vi "Sample_process.vi"(8 "Start":i32=20, 9 "Frame number":i32, 11 "Sample data":dbl[](array[numeric])) -> (3 "Image date":dbl[](array[numeric]))   [LabVIEW 2016]
uses:
  <vilib>/Analysis/baseanly.llb/Mean (DBL).vi
  <vilib>/Analysis/NI_AALBase.lvlib
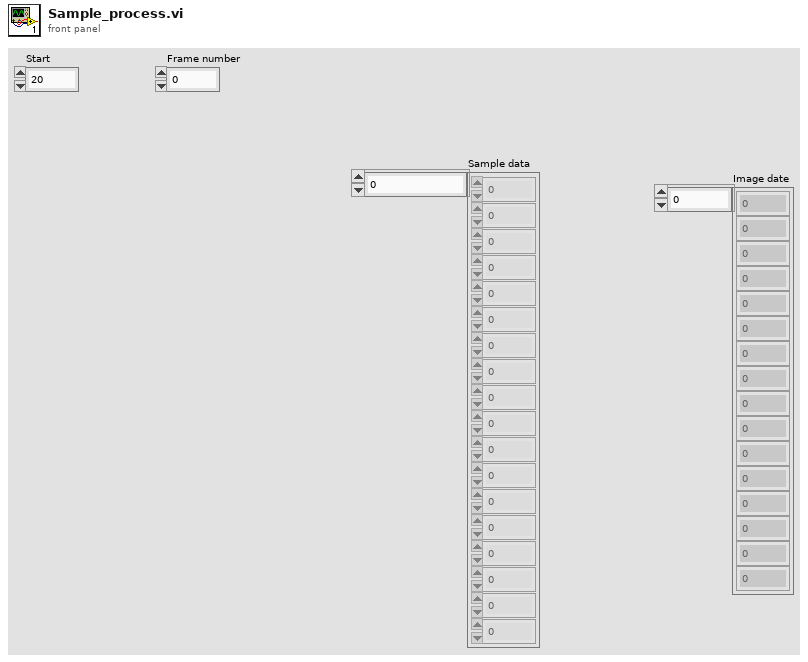
[diagram p1: front panel]
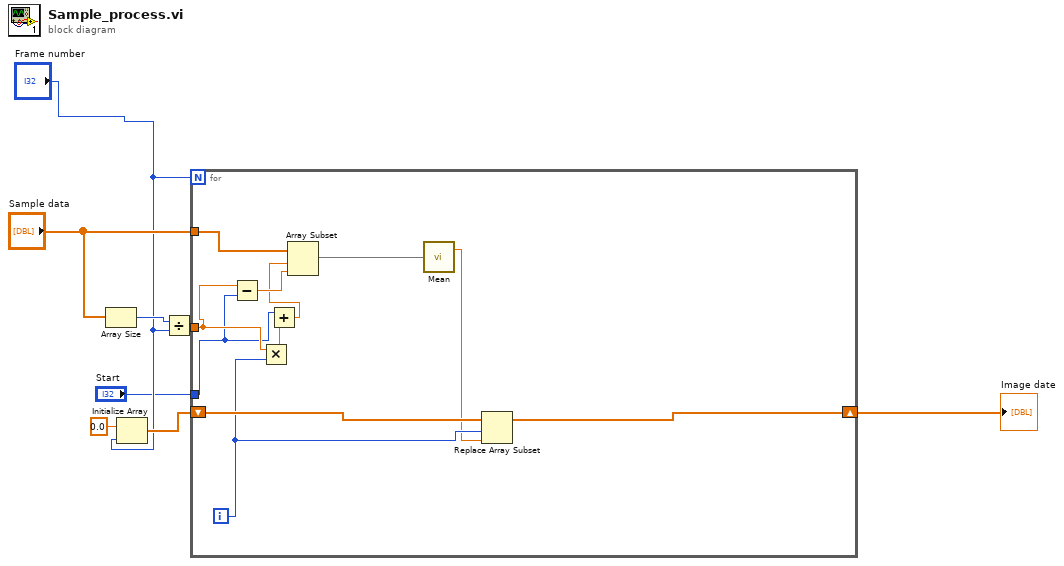
[diagram p0: block diagram]
diagram:
  n1 = Array Size(array="Sample data") -> (size(s)=w7:i32)
  n2 = Initialize Array(0.0 ("element"), "Frame number") -> (w4:dbl[])
  n3 = Divide(x=w7, y="Frame number") -> (x/y=w6:dbl)
  n4 = for {
    N: "Frame number" -> [_]
    tunnel: "Sample data" -> [w19]
    tunnel: w6 -> [w12]
    shift-right: [w16] -> w3
    shift-left: w4 -> [w17]
    tunnel: "Start" -> [w11]
    i -> [w15]
    n5 = Subtract(x=w12, y=w11) -> (x-y=w10:dbl)
    n6 = Multiply(x=w12, y=w15) -> (x*y=w18:dbl)
    n7 = Add(x=w11, y=w18) -> (x+y=w9:dbl)
    n8 = Array Subset(array=w19, index=w9, length=w10) -> (w14:dbl[])
    n9 = call-poly <vilib>:"Mean.vi"("X"=w14) -> ("mean"=w13:dbl)  [unwired: 1 out]
    n10 = Replace Array Subset(array=w17, new element=w13, index=w15) -> (w16:dbl[])
  }
  "Image date" <- w3
